vi "Read Coms from Drone.vi"() -> ()   [LabVIEW 2014]
uses:
  Controls/MAVLink Packet.ctl
  Controls/MAVLink Heartbeat.ctl
  Controls/MAVLink System Status.ctl
  Aircraft Information/Controls/Aircraft Sensor Status Data.ctl
  GUI Design/Indicators/Sensor Status LED CLuster.ctl
  GUI Design/Indicators/Status LED.ctl
panel:
  out "Aircraft System Status Out":T1 {"Communication Drop Rate (%)" scale=0.0..100.0; "Battery Remaining (%)" scale=0.0..100.0; "CPU Load (%)" scale=0.0..100.0}
  out "output cluster":T4
  out "System Status":T5
  out "Heartbeat":T6 {"custom_mode" format="%x"}
  out "Packet":T7
  out "address":u32
  out "port":u16
  out "Numeric Control":i32
  out "error out":errorcluster
  in  "error in (no error)":errorcluster
  in  "Stop":bool
  out "data out":string
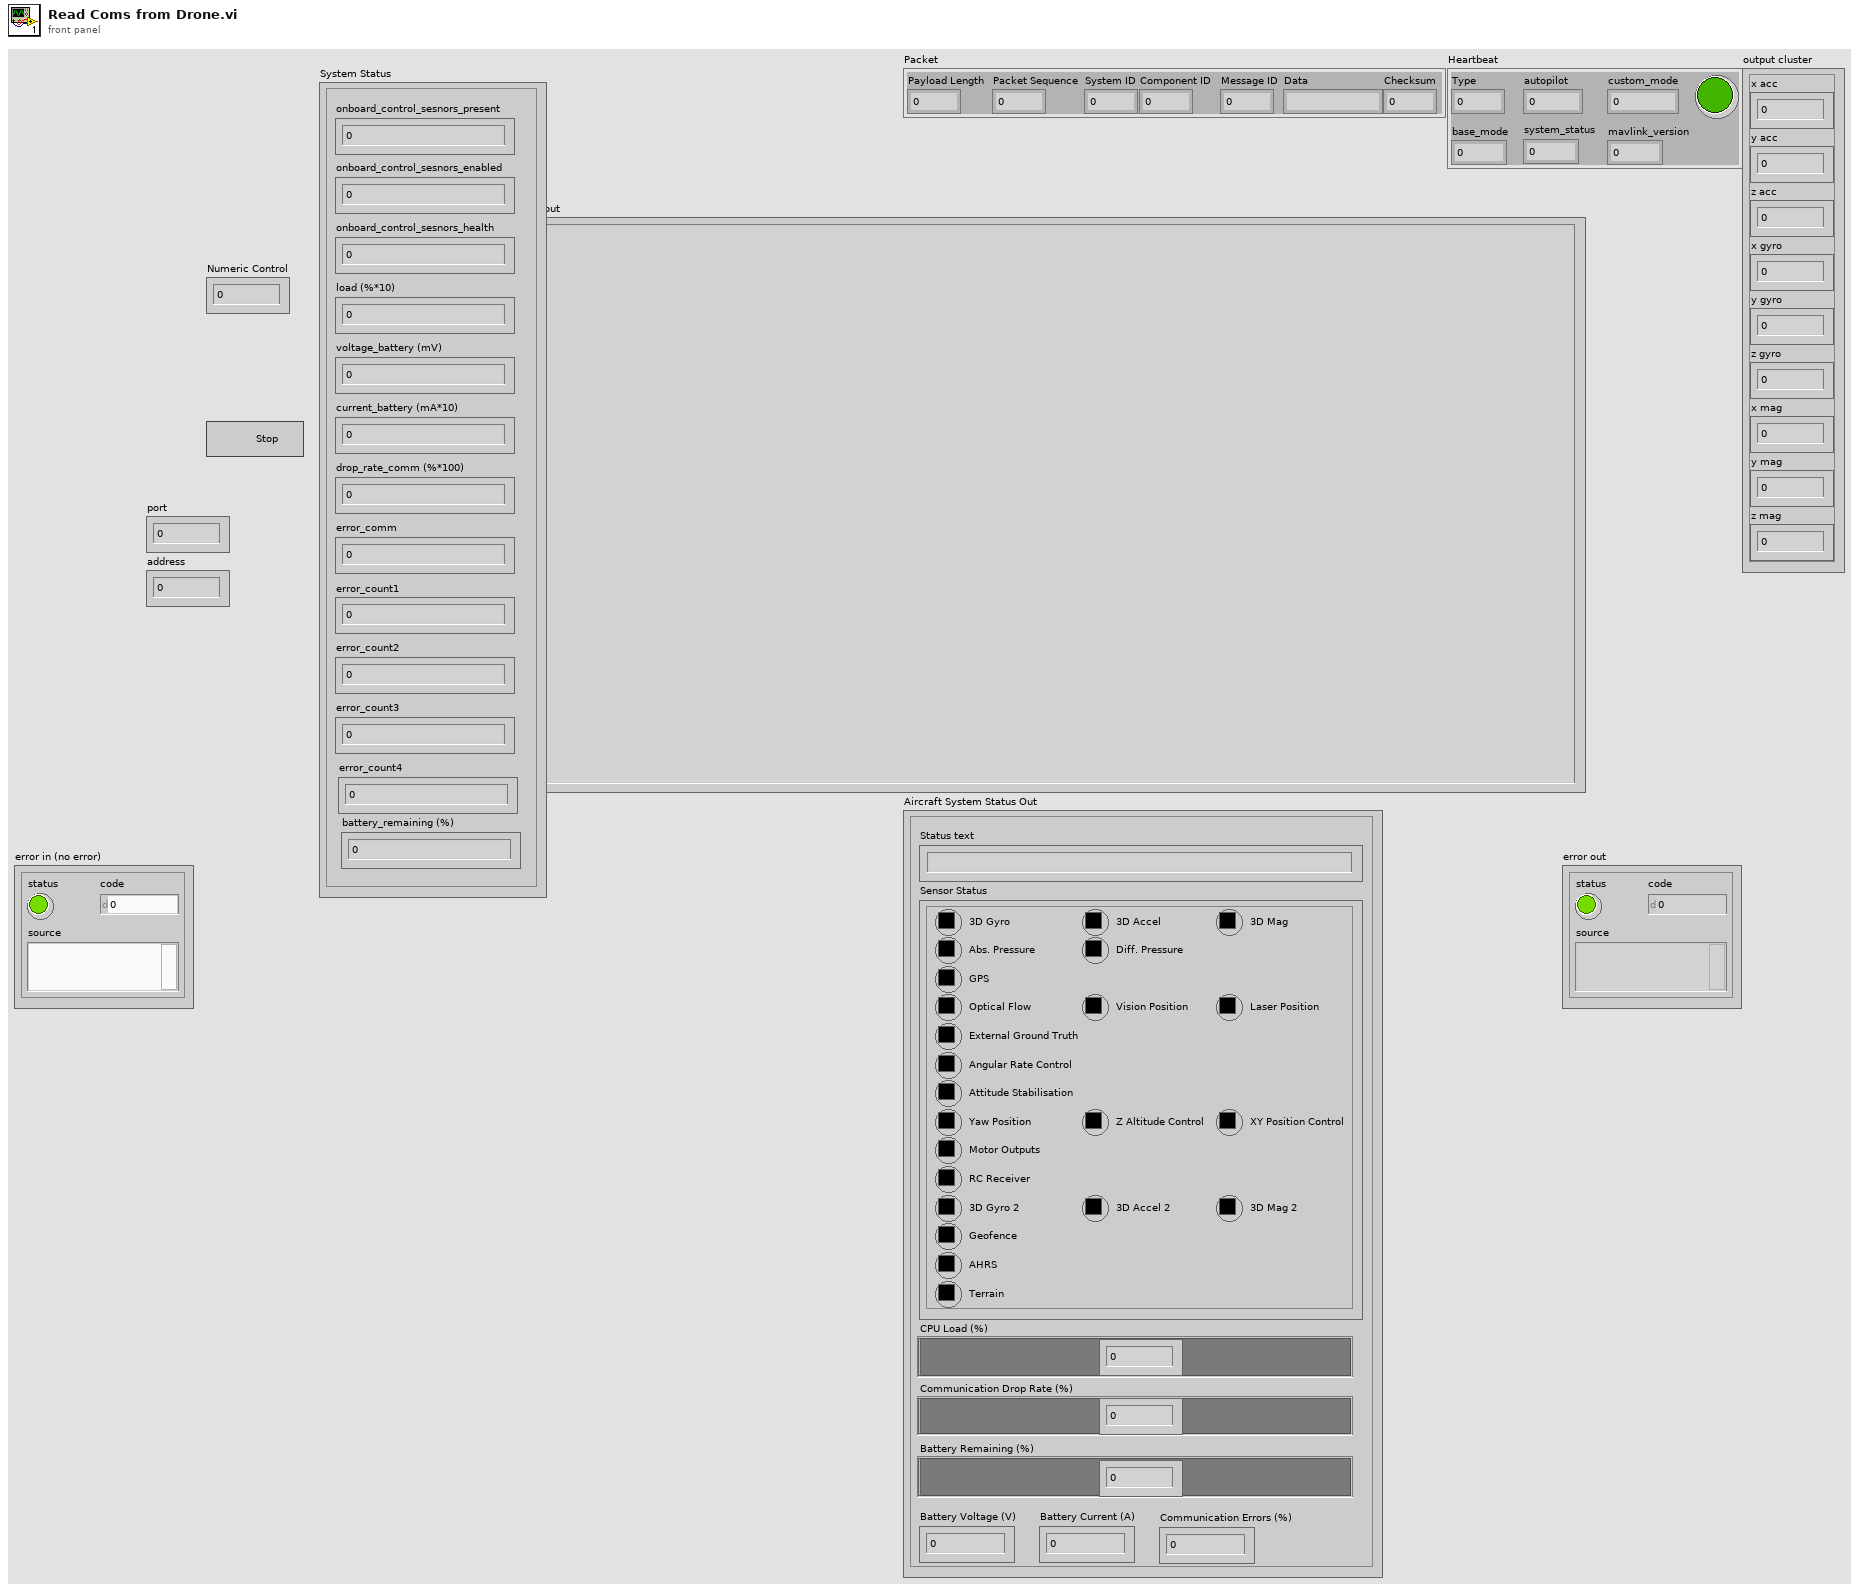
[diagram p1: front panel]
types:
  T1 = typedef "Aircraft Sensor Status Data.ctl" = cluster{"Sensor Status":T2, "CPU Load (%)":dbl, "Battery Voltage (V)":dbl, "Battery Current (A)":dbl, "Battery Remaining (%)":dbl, "Communication Drop Rate (%)":dbl, "Communication Errors (%)":dbl, "Status text":string}
  T2 = typedef "Sensor Status LED CLuster.ctl" = cluster{"3D Gyro":u32, "3D Accel":u32, "3D Mag":u32, "Abs. Pressure":u32, "Diff. Pressure":u32, "GPS":T3, "Optical Flow":u32, "Vision Position":u32, "Laser Position":u32, "External Ground Truth":u32, "Angular Rate Control":u32, "Attitude Stabilisation":u32, "Yaw Position":u32, "Z Altitude Control":u32, "XY Position Control":u32, "Motor Outputs":u32, "RC Receiver":u32, "3D Gyro 2":u32, "3D Accel 2":u32, "3D Mag 2":u32, "Geofence":u32, "AHRS":u32, "Terrain":u32}
  T3 = typedef "Status LED.ctl" = u32
  T4 = cluster{"x acc":i16, "y acc":i16, "z acc":i16, "x gyro":i16, "y gyro":i16, "z gyro":i16, "x mag":i16, "y mag":i16, "z mag":i16}
  T5 = typedef "MAVLink System Status.ctl" = cluster{"onboard_control_sesnors_present":u32, "onboard_control_sesnors_enabled":u32, "onboard_control_sesnors_health":u32, "load (%*10)":u16, "voltage_battery (mV)":u16, "current_battery (mA*10)":i16, "drop_rate_comm (%*100)":u16, "error_comm":u16, "error_count1":u16, "error_count2":u16, "error_count3":u16, "error_count4":u16, "battery_remaining (%)":i8}
  T6 = typedef "MAVLink Heartbeat.ctl" = cluster{"custom_mode":u32, "Type":u8, "autopilot":u8, "base_mode":u8, "system_status":u8, "mavlink_version":u8, "heartbeat":bool}
  T7 = typedef "MAVLink Packet.ctl" = cluster{"Payload Length":u8, "Packet Sequence":u8, "System ID":u8, "Component ID":u8, "Message ID":u8, "Data":string, "Checksum":u16}
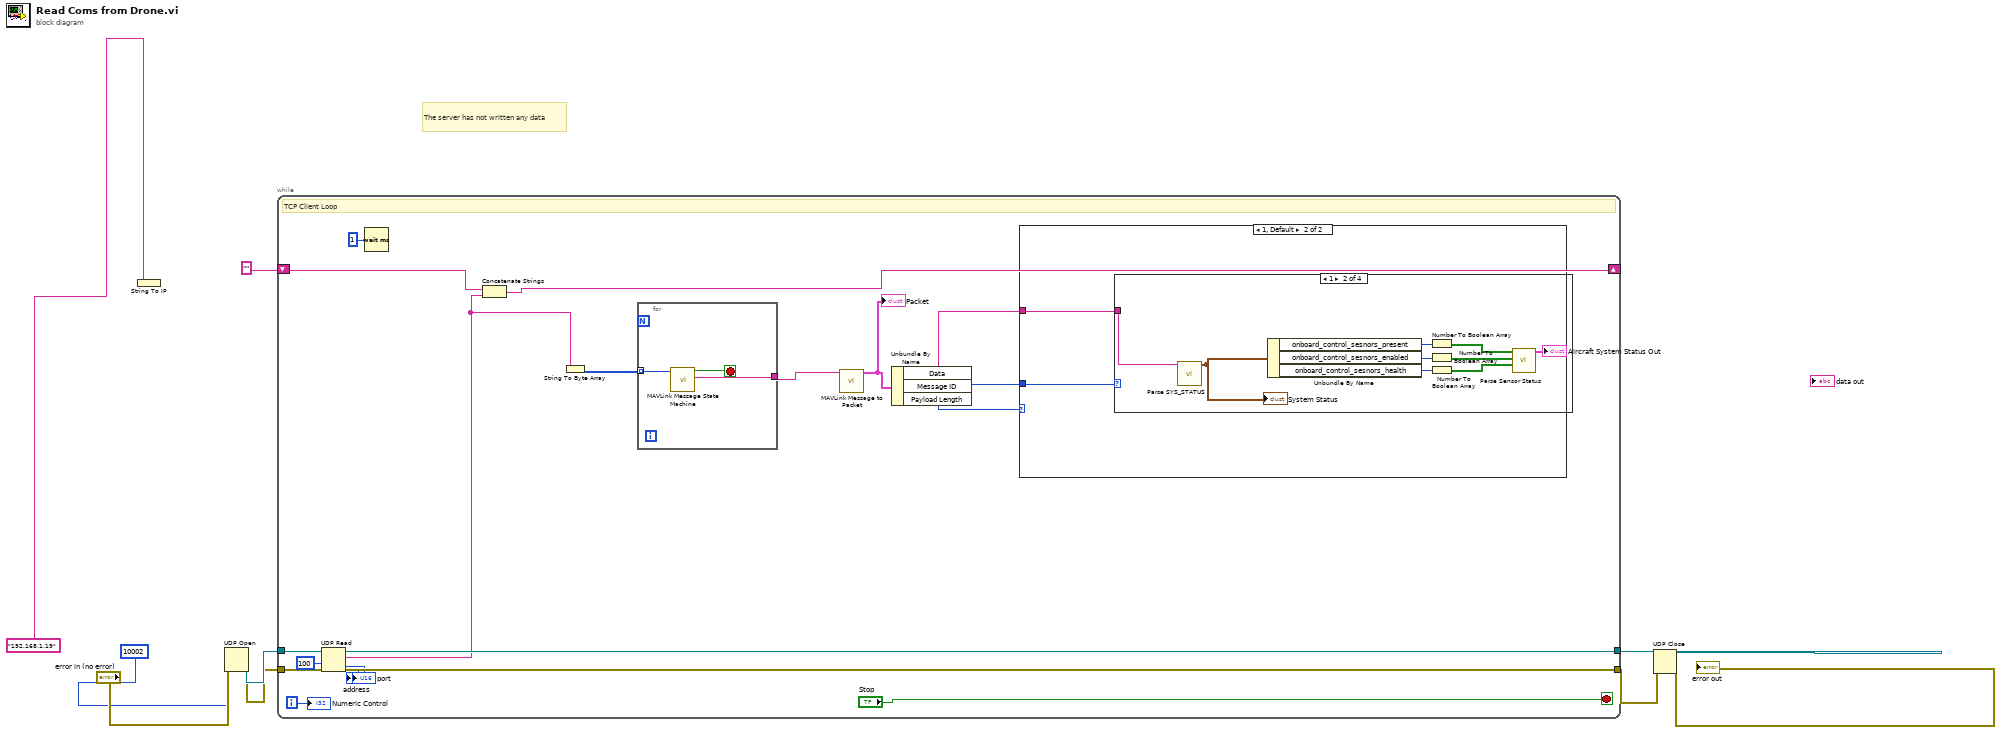
[diagram p0: block diagram]
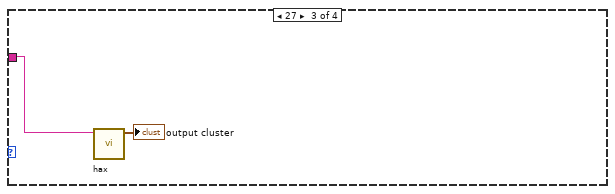
[diagram p4: hidden frame]
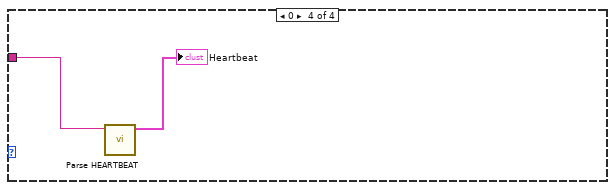
[diagram p5: hidden frame]
diagram:
  # "The server has not written any data"
  n1 = String To IP(1:"192.168.1.19" ("address")) -> ()  [unwired: 1 out]
  n2 = UDP Open(8:"error in (no error)", 11:u16 10002 ("remote port or service name")) -> (port=w9:refnum<k16>, 0:w8:errorcluster)  [unwired: 3 in, 1 out]
  n3 = while {
    tunnel: w8 -> [w22]
    tunnel: w9 -> [w23]
    tunnel: [w21] -> w3
    tunnel: [w20] -> w4
    shift-right: [w27] -> _
    shift-left: "" -> [w26]
    i -> [w25]
    stop <- "Stop" stop-if-true
    # "TCP Client Loop"
    n4 = UDP Read(connection ID=w23, timeout ms (25000)=100, 8:w22) -> (data out=w16:string, error out=w20:errorcluster, 3:w21:refnum<k16>, 4:→"port":u16, 6:→"address":u32)  [unwired: 1 in]
    n5 = Wait (ms)(milliseconds to wait=u32 1) -> ()  [unwired: 1 out]
    n6 = Concatenate Strings(w26, w16) -> (w27:string)
    n7 = String To Byte Array(string=w16) -> (unsigned byte array=w15:u8[])
    n8 = for {
      tunnel: w15 -> [w46] mode=indexing
      tunnel: [w44] -> w14
      stop <- w45 stop-if-true
      n9 = call "MAVLink Message State Machine.vi"("Incoming Bytes"=w46) -> ("Message"=w44:string, "Message Complete"=w45:bool)  [unwired: 8 in, 1 out]
    }
    n10 = call "MAVLink Message to Packet.vi"("Message"=w14) -> ("Packet"=w13:T7)  [unwired: 10 in]
    "Packet" <- w13
    n11 = Unbundle By Name(w13) -> ("Data"=w12:string, "Message ID"=w11:u8, "Payload Length"=w10:u8)
    n12 = case shown="1, Default" w10 {
      tunnel: w12 -> [_ w30]
      tunnel: w11 -> [_ w29]
      frame 0 {
      }
      frame 1, Default {
        n13 = case shown="1" w29 {
          tunnel: w30 -> [_ w39 w41 w43]
          frame 2, Default {
          }
          frame 1 {
            n14 = call "Parse SYS_STATUS.vi"("Data"=w39) -> ("System Status"=w32:T5)  [unwired: 10 in]
            "System Status" <- w32
            n15 = Unbundle By Name(w32) -> ("onboard_control_sesnors_present"=w35:u32, "onboard_control_sesnors_enabled"=w34:u32, "onboard_control_sesnors_health"=w33:u32)
            n16 = Number To Boolean Array(number=w35) -> (Boolean array=w38:bool[])
            n17 = Number To Boolean Array(number=w34) -> (Boolean array=w37:bool[])
            n18 = Number To Boolean Array(number=w33) -> (Boolean array=w36:bool[])
            n19 = call "Parse Sensor Status.vi"("Healthy"=w36, "Enabled"=w37, "Present"=w38) -> ("Aircraft System Status Out"=→"Aircraft System Status Out":T1)  [unwired: 8 in]
          }
          frame 27 {
            n20 = call "hax.vi"("string"=w41) -> ("output cluster"=→"output cluster":T4)  [unwired: 10 in]
          }
          frame 0 {
            n21 = call "Parse HEARTBEAT.vi"("Data"=w43) -> ("Heartbeat"=→"Heartbeat":T6)  [unwired: 10 in]
          }
        }
      }
    }
    "Numeric Control" <- w25
  }
  n22 = UDP Close(connection ID=w3, 8:w4) -> (error out=→"error out":errorcluster)  [unwired: 1 out]
